vi "Prepare Config Files.vi"(8 "error in":errorcluster, 10 "Config Prefix":string, 11 "Project Root":path) -> (0 "error out":errorcluster, 2 "Log Directory":path, 3 "Config Directory":path)   [LabVIEW 2011]
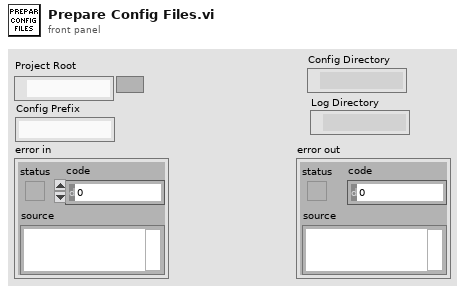
[diagram p1: front panel]
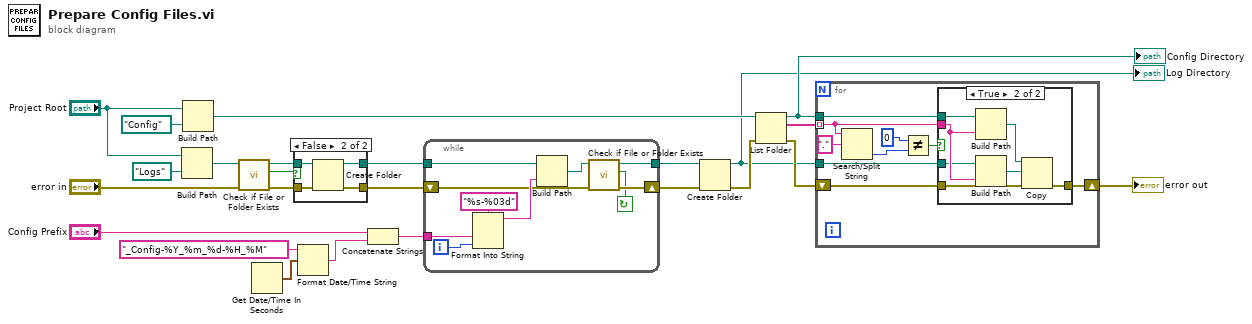
[diagram p0: block diagram]
diagram:
  n1 = Build Path(base path="Project Root", name or relative path=path "Logs") -> (appended path=w21:path)
  n2 = Build Path(base path="Project Root", name or relative path=path "Config") -> (appended path=w6:path)
  n3 = call <vilib>:"Check if File or Folder Exists.vi"("error in (no error)"="error in", "path"=w21) -> ("error out"=w19:errorcluster, "file or folder exists?"=w17:bool, "dup path"=w18:path)  [unwired: 7 in]
  n4 = Get Date/Time In Seconds() -> (seconds since 1Jan1904=w23:timestamp)
  n5 = case shown="False" w17 {
    tunnel: [w26 w30] -> w15
    tunnel: [w25 w29] -> w16
    tunnel: w19 -> [w25 w28]
    tunnel: w18 -> [w26 w27]
    frame True {
    }
    frame False {
      n6 = Create Folder(path (use dialog)=w27, error in=w28) -> (created path=w30:path, error out=w29:errorcluster)  [unwired: 1 in, 1 out]
    }
  }
  n7 = Format Date/Time String(time format string (%c)="_Config-%Y_%m_%d-%H_%M", seconds (now)=w23) -> (date/time string=w5:string)  [unwired: 1 in]
  n8 = Concatenate Strings("Config Prefix", w5) -> (w4:string)
  n9 = while {
    tunnel: w15 -> [w37]
    tunnel: w4 -> [w38]
    shift-right: [w33] -> w14
    shift-left: w16 -> [w34]
    tunnel: [w31] -> w13
    i -> [w39]
    stop <- w32 continue-if-true
    n10 = Format Into String(format string="%s-%03d", w38, w39) -> (resulting string=w36:string)  [unwired: 2 in, 1 out]
    n11 = Build Path(base path=w37, name or relative path=w36) -> (appended path=w35:path)
    n12 = call <vilib>:"Check if File or Folder Exists.vi"("error in (no error)"=w34, "path"=w35) -> ("error out"=w33:errorcluster, "file or folder exists?"=w32:bool, "dup path"=w31:path)  [unwired: 7 in]
  }
  n13 = Create Folder(path (use dialog)=w13, error in=w14) -> (created path=w1:path, error out=w12:errorcluster)  [unwired: 1 in, 1 out]
  "Log Directory" <- w1
  n14 = List Folder(path=w6, error in=w12) -> (path out=w2:path, filenames=w11:string[], error out=w10:errorcluster)  [unwired: 2 in, 1 out]
  "Config Directory" <- w2
  n15 = for {
    tunnel: w11 -> [w45] mode=indexing
    tunnel: w2 -> [w49]
    tunnel: w1 -> [w46]
    shift-right: [w47] -> w9
    shift-left: w10 -> [w48]
    n16 = Search/Split String(string=w45, search string/char (-)=".") -> (offset of match=w42:i32)  [unwired: 1 in, 2 out]
    n17 = Not Equal?(x=0, y=w42) -> (x != y?=w43:bool)
    n18 = case shown="True" w43 {
      tunnel: w49 -> [_ w57]
      tunnel: w45 -> [_ w56]
      tunnel: w48 -> [w50 w55]
      tunnel: [w50 w52] -> w47
      tunnel: w46 -> [_ w51]
      frame False {
      }
      frame True {
        n19 = Build Path(base path=w57, name or relative path=w56) -> (appended path=w54:path)
        n20 = Build Path(base path=w51, name or relative path=w56) -> (appended path=w53:path)
        n21 = Copy(8:w55, 10:w53, 11:w54) -> (0:w52:errorcluster)  [unwired: 2 in, 2 out]
      }
    }
  }
  "error out" <- w9
